vi "toString.vi"(8 "error in (no error)":errorcluster, 11 "NativeXML in":refnum<class "NativeXML.lvclass">) -> (0 "error out":errorcluster, 2 "xmlString":string, 3 "NativeXML out":refnum<class "NativeXML.lvclass">)   [LabVIEW 2009, in "Tools.lvlib" / "xml.lvlib" / "NativeXML.lvclass"]
uses:
  NativeXML.lvclass
  NativeXML.lvclass/NativeXML.ctl
  Program Files/National Instruments/LabVIEW 2009/resource/objmgr/DOMUserDefRef.rc
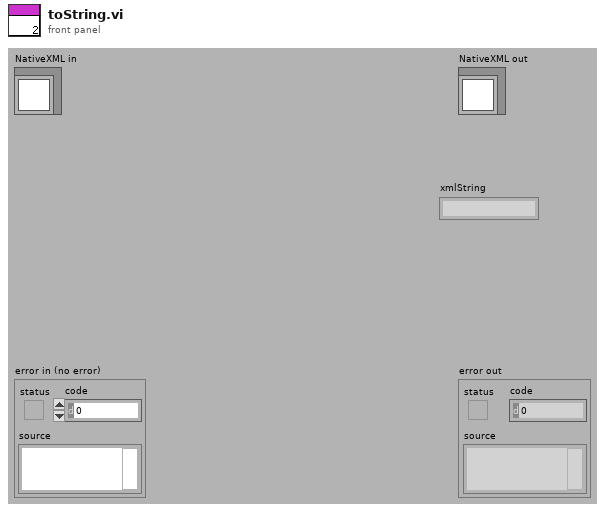
[diagram p1: front panel]
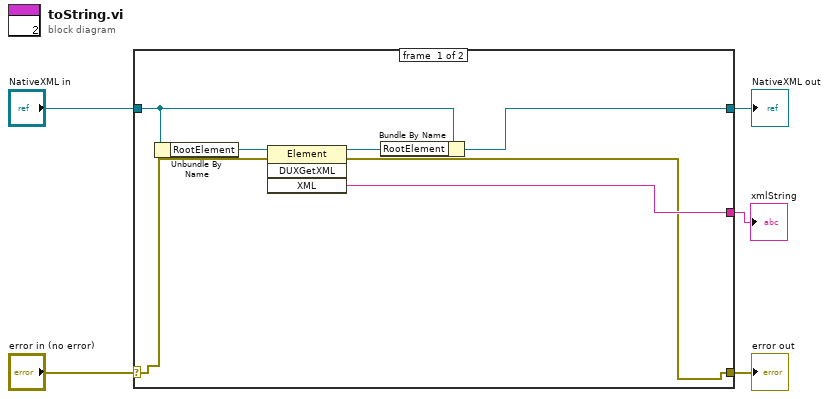
[diagram p0: block diagram]
diagram:
  n1 = case shown="No Error" "error in (no error)" {
    selector: "error in (no error)" -> [w9 w14]
    tunnel: [w7 w14] -> w4
    tunnel: [w11 w13] -> w2
    tunnel: "NativeXML in" -> [w12 w13]
    tunnel: [w8 _] -> w1
    frame #0 {
      n2 = Unbundle By Name(w12) -> ("RootElement"=w10:refnum<k20>)
      n3 = invoke class="Element" method="DUXGetXML"(reference=w10, error in=w9) -> (reference out=w6:refnum<k20>, error out=w7:errorcluster, "XML"=w8:string)  [unwired: 2 in, 1 out]
      n4 = Bundle By Name(cluster=w12, "RootElement"=w6) -> (w11:refnum<class "NativeXML.lvclass">)
    }
    frame #1 {
    }
  }
  "error out" <- w4
  "NativeXML out" <- w2
  "xmlString" <- w1
